vi "PPFS_SIM_Gyro_Read.vi"(9 "GyroDevRef":T1) -> (1 "Gyro_Cont_Deg":dbl)   [LabVIEW 2023]
uses:
  <vilib>/Rock Robotics/WPI/ThirdParty/Phoenix6/getters/GetPigeon2Yaw.vi
  <vilib>/Rock Robotics/WPI/ThirdParty/Phoenix6/DeviceReference.ctl
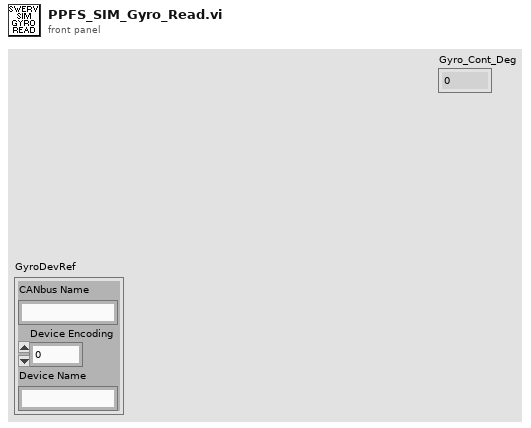
[diagram p1: front panel]
types:
  T1 = typedef "DeviceReference.ctl" = cluster{"CANbus Name":string, "Device Encoding":u32, "Device Name":string}
  T2 = cluster{"Value":dbl, "System Timestamp":dbl, "CANivore Timestamp":dbl, "ECU Timestamp":dbl}
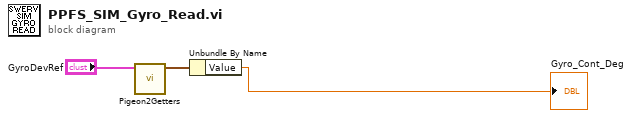
[diagram p0: block diagram]
diagram:
  n1 = call-poly <vilib>:"Pigeon2Getters.vi"("DeviceReference"="GyroDevRef") -> ("Output"=w2:T2)  [unwired: 9 in, 1 out]
  n2 = Unbundle By Name(w2) -> ("Value"=→"Gyro_Cont_Deg":dbl)
